vi "MySQL_Open_DB.vi"(7 "Connected? in":refnum<vi>, 8 "Status/Errors in":refnum<vi>, 9 "Password":string, 10 "User":string, 11 "DB name":string) -> (0 "Status/Errors out":refnum<vi>, 2 "DB connection":T1)   [LabVIEW 2010]
doc: "Tries to open a connection with the local MySQL database. Returns a cluster \"DB connection\" that consists of a boolean \"Connected?\" together with a reference to the database connection."
uses:
  Controls/DB_Connection.ctl
  database/Connection.llb/Conn ObjectReference.ctl
  Controls/Get_Set_Statistics_Options2.ctl
  Controls/Master.ctl
  database/Connection.llb/DB Tools Open Connec (String).vi
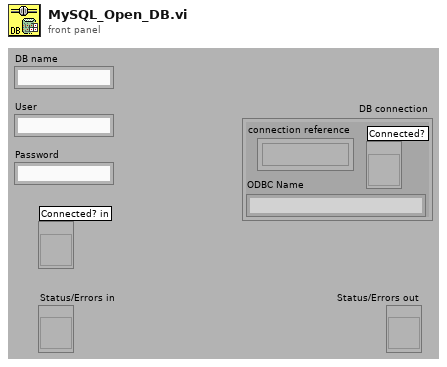
[diagram p1: front panel]
types:
  T1 = typedef "DB_Connection.ctl" = cluster{"connection reference":T2, "Connected?":refnum<vi>, "ODBC Name":string}
  T2 = typedef "Conn ObjectReference.ctl" = refnum<k1>
  T3 = typedef "Get_Set_Statistics_Options2.ctl" = enum16{"Get", "Set"}
  T4 = typedef "Master.ctl" = enum16{"Master", "Slave", "General"}
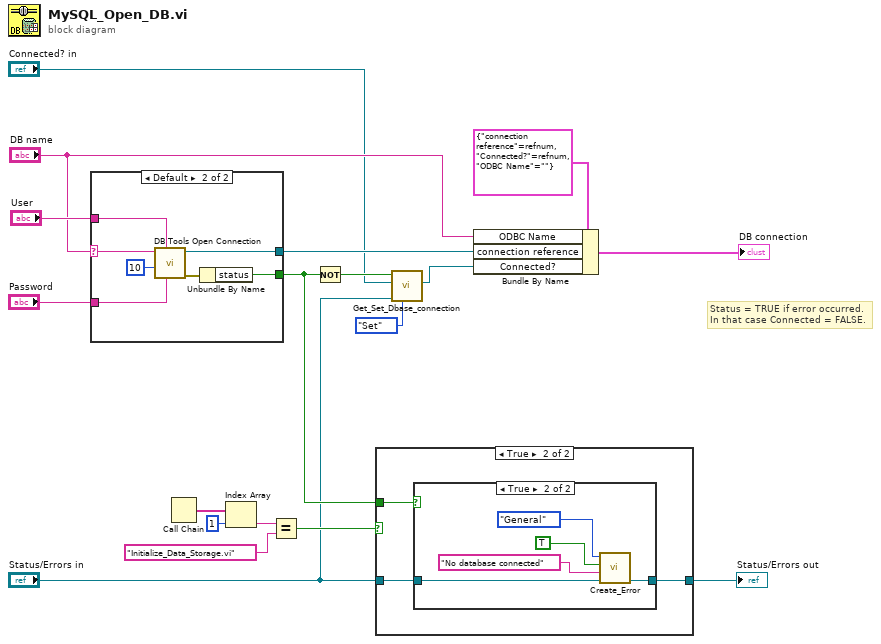
[diagram p0: block diagram]
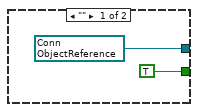
[diagram p2: hidden frame]
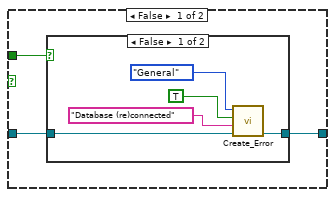
[diagram p3: hidden frame]
diagram:
  # "Status = TRUE if error occurred.\nIn that case Connected = FALSE."
  n1 = case shown="Default" "DB name" {
    selector: "DB name" -> [_ w21]
    tunnel: "User" -> [_ w27]
    tunnel: "Password" -> [_ w26]
    tunnel: [w19 w25] -> w14
    tunnel: [TRUE ("status") w22] -> w8
    frame "" {
      w19 = T2 refnum items=["Connection"] ("connection reference")
    }
    frame Default {
      n2 = call-poly "DB Tools Open Connection.vi"("password"=w26, "userID"=w27, "connection timeout (15)"=10, "connection information"=w21) -> ("error out"=w24:errorcluster, "connection reference"=w25:T2)  [unwired: 2 in, 2 out]
      n3 = Unbundle By Name(w24) -> ("status"=w22:bool)
    }
  }
  n4 = Call Chain() -> (call chain=w12:string[])
  n5 = Index Array(array=w12, index=1) -> (element=w10:string)
  n6 = Equal?(x=w10, y="Initialize_Data_Storage.vi") -> (x = y?=w6:bool)
  n7 = Not(x=w8) -> (.not. x?=w5:bool)
  n8 = case shown="True" w6 {
    tunnel: "Status/Errors in" -> [w29 w38]
    tunnel: [w30 w39] -> w13
    tunnel: w8 -> [w28 w37]
    frame False {
      n9 = case shown="False" w28 {
        tunnel: [w35 w36] -> w30
        tunnel: w29 -> [w34 w36]
        frame False {
          n10 = call "Create_Error.vi"("Status/Errors in"=w34, "HiSPARC error"="Database (re)connected" ("error message (\"\")"), "Warning? (false)"=TRUE, "Master?"=Master."General") -> ("Status/Errors out"=w35:refnum<vi>)  [unwired: 2 in, 5 out]
        }
        frame True {
        }
      }
    }
    frame True {
      n11 = case shown="True" w37 {
        tunnel: [w40 w45] -> w39
        tunnel: w38 -> [w40 w44]
        frame False {
        }
        frame True {
          n12 = call "Create_Error.vi"("Status/Errors in"=w44, "HiSPARC error"="No database connected" ("error message (\"\")"), "Warning? (false)"=TRUE, "Master?"=Master."General") -> ("Status/Errors out"=w45:refnum<vi>)  [unwired: 2 in, 5 out]
        }
      }
    }
  }
  "Status/Errors out" <- w13
  n13 = call "Get_Set_Dbase_connection.vi"("Get/Set"=Get_Set_Statistics_Options2."Set", "Status/Errors in"="Status/Errors in", "Connected? in"="Connected? in", "Value in"=w5) -> ("Connected? out"=w4:refnum<vi>)  [unwired: 7 out]
  n14 = Bundle By Name(cluster=T1 {"connection reference"=refnum, "Connected?"=refnum, "ODBC Name"=""} ("DB connection"), "ODBC Name"="DB name", "connection reference"=w14, "Connected?"=w4) -> (→"DB connection":T1)
